vi "Nonlinear Curve Fit Intervals (Pearson option).vi"(0 "Y":dbl[](array[numeric]), 1 "confidence level":dbl=0.95, 2 "f(x,a)":T1, 3 "data":variant, 5 "X":dbl[](array[numeric]), 7 "Weight":dbl[](array[numeric]), 9 "best fit parameters":dbl[](array[numeric]), 11 "error in (no error)":errorcluster) -> (4 "Upper Bound":dbl[](array[numeric]), 6 "Lower Bound":dbl[](array[numeric]), 10 "delta best fit parameters":dbl[](array[numeric]), 15 "error out":errorcluster)   [LabVIEW 2021, in "Fits.lvlib"]
doc: "Calculates statistical intervals of the best nonlinear fit for a data set (<B>X</B>, <B>Y</B>)."
uses:
  <vilib>/gmath/NumericalOptimization/LM model function reference.ctl
  <vilib>/gmath/NumericalOptimization/LM_output select.ctl
  <vilib>/Analysis/baseanly.llb/Real A x B.vi
  <vilib>/gmath/statdist.llb/Student t Inverse CDF.vi
  <vilib>/Analysis/baseanly.llb/Real Inverse Matrix.vi
  Fits.lvlib
  <vilib>/Analysis/NI_AALPro.lvlib
  <vilib>/gmath/NI_Gmath.lvlib
  <vilib>/Analysis/NI_AALBase.lvlib
panel:
  # "see the License on the block diagram (Ctrl+E or Window:Show Block Diagram)"
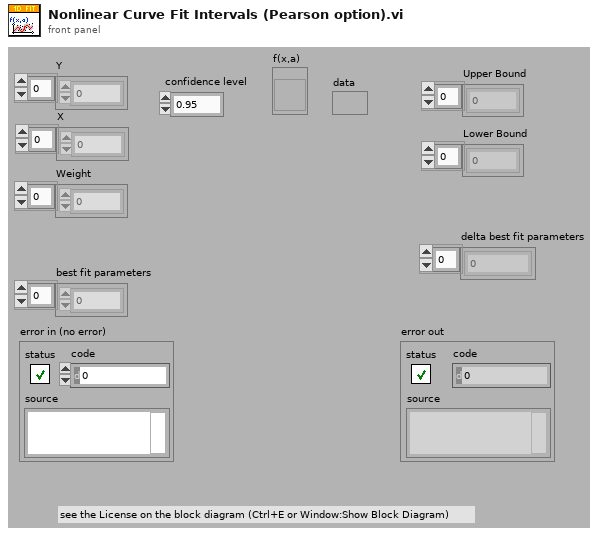
[diagram p1: front panel]
types:
  T1 = typedef "NI_Gmath.lvlib/LM model function reference.ctl" = refnum<vi>
  T2 = typedef "NI_Gmath.lvlib/LM_output select.ctl" = cluster{"model function":bool, "gradient":bool}
  T3 = typedef "NI_Matrix.lvlib/RealMatrix.ctl" = dbl[][]
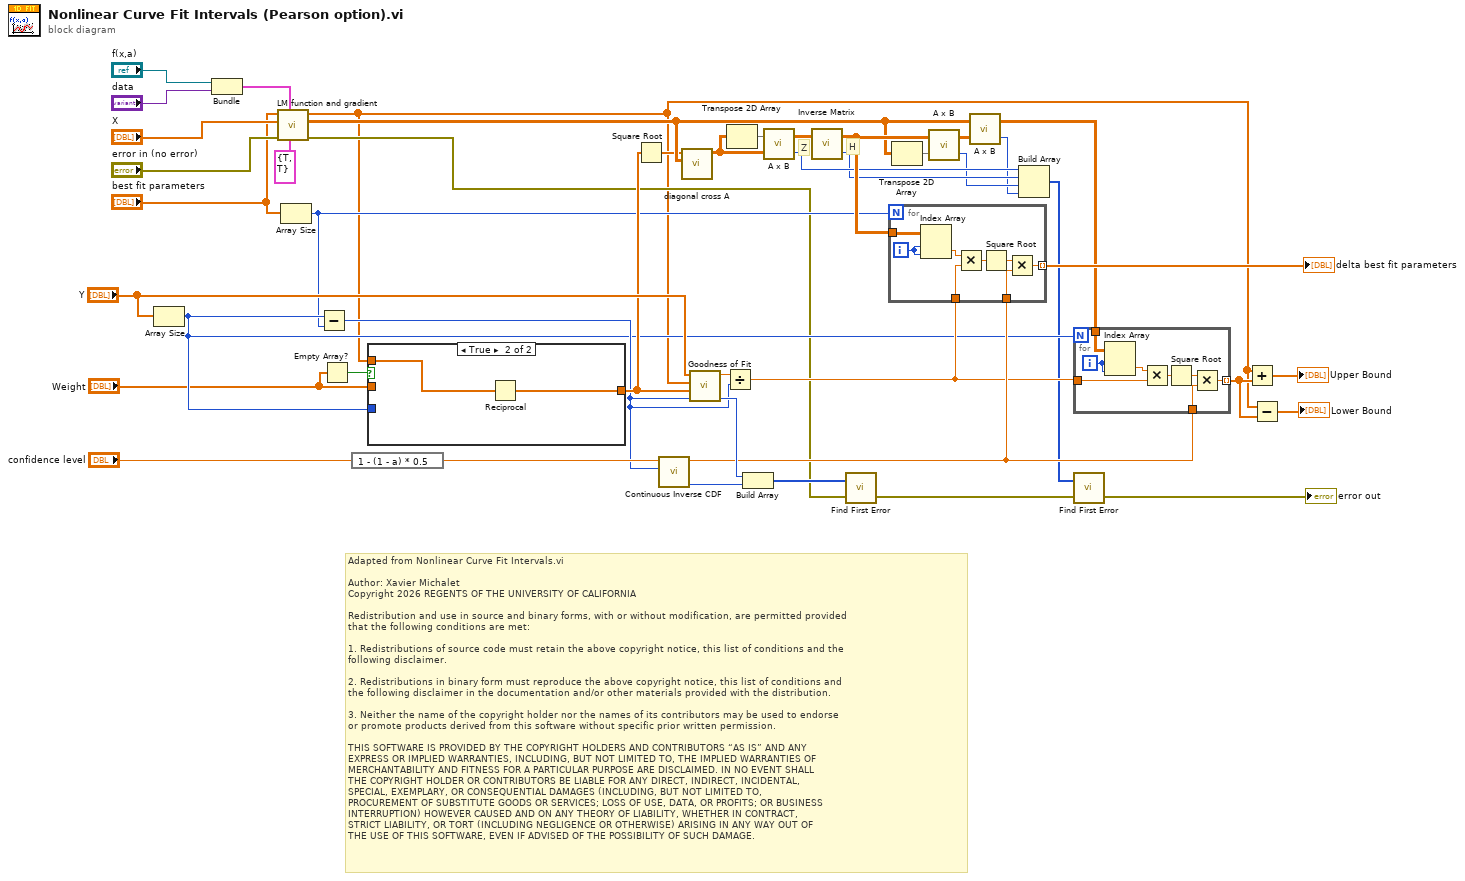
[diagram p0: block diagram]
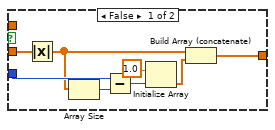
[diagram p2: hidden frame]
diagram:
  # "Adapted from Nonlinear Curve Fit Intervals.vi\n\nAuthor: Xavier Michalet\nCopyright 2026 REGENTS OF THE UNIVERSITY OF CALIFORNIA\n\nRedistribution and use in source and binary forms, with or without modification, are permitted provided\nthat the following conditions are met:\n\n1. Redistributions of source code must retain the above copyright notice, this list of conditions and the\nfollowing disclaimer.\n\n2. Redistributions in binary form must reproduce the above copyright notice, this list of conditions and\nthe following disclaimer in the documentation and/or other materials provided with the distribution.\n\n3. Neither the name of the copyright holder nor the names of its contributors may be used to endorse \nor promote products derived from this software without specific prior written permission.\n\nTHIS SOFTWARE IS PROVIDED BY THE COPYRIGHT HOLDERS AND CONTRIBUTORS “AS IS” AND ANY \nEXPRESS OR IMPLIED WARRANTIES, INCLUDING, BUT NOT LIMITED TO, THE IMPLIED WARRANTIES OF\nMERCHANTABILITY AND FITNESS FOR A PARTICULAR PURPOSE ARE DISCLAIMED. IN NO EVENT SHALL\nTHE COPYRIGHT HOLDER OR CONTRIBUTORS BE LIABLE FOR ANY DIRECT, INDIRECT, INCIDENTAL, \nSPECIAL, EXEMPLARY, OR CONSEQUENTIAL DAMAGES (INCLUDING, BUT NOT LIMITED TO, \nPROCUREMENT OF SUBSTITUTE GOODS OR SERVICES; LOSS OF USE, DATA, OR PROFITS; OR BUSINESS\nINTERRUPTION) HOWEVER CAUSED AND ON ANY THEORY OF LIABILITY, WHETHER IN CONTRACT, \nSTRICT LIABILITY, OR TORT (INCLUDING NEGLIGENCE OR OTHERWISE) ARISING IN ANY WAY OUT OF\nTHE USE OF THIS SOFTWARE, EVEN IF ADVISED OF THE POSSIBILITY OF SUCH DAMAGE."
  # "H"
  # "Z"
  n1 = Array Size(array="Y") -> (size(s)=w16:i32)
  n2 = Bundle("f(x,a)"="f(x,a)", "data"="data") -> (w40:cluster{"f(x,a)":T1, "data":variant})  [unwired: 1 in]
  n3 = call <vilib>:"LM function and gradient.vi"("output control"=T2 {"model function"=TRUE, "gradient"=TRUE}, "model function"=w40, "error in (no error)"="error in (no error)", "X"="X", "a"="best fit parameters") -> ("error out"=w7:errorcluster, "gradient"=w6:dbl[][], "f(X)"=w1:dbl[])  [unwired: 3 in, 1 out]
  n4 = Array Size(array="best fit parameters") -> (size(s)=w15:i32)
  n5 = Subtract(x=w16, y=w15) -> (x-y=w17:i32)
  n6 = Empty Array?(array="Weight") -> (empty?=w2:bool)
  n7 = expression code="1 - (1 - a) * 0.5"("confidence level") -> (w30:dbl)
  n8 = case shown="True" w2 {
    tunnel: "Weight" -> [w48 _]
    tunnel: [w47 w53] -> w18
    tunnel: w16 -> [w46 _]
    tunnel: w1 -> [_ w54]
    frame False {
      n9 = Absolute Value(x=w48) -> (abs(x)=w45:dbl[])
      n10 = Array Size(array=w45) -> (size(s)=w51:i32)
      n11 = Subtract(x=w46, y=w51) -> (x-y=w49:i32)
      n12 = Initialize Array(1.0, w49) -> (w50:dbl[])
      n13 = Build Array (concatenate)(w45, w50) -> (w47:dbl[])
    }
    frame True {
      n14 = Reciprocal(x=w54) -> (1/x=w53:dbl[])
    }
  }
  n15 = Square Root(x=w18) -> (sqrt(x)=w5:dbl[])
  n16 = call-poly <vilib>:"Continuous Inverse CDF.vi"("k degrees of freedom"=w17, "cdf(x)"=w30) -> ("error"=w29:i32, "x"=w24:dbl)  [unwired: 8 in]
  n17 = call <vilib>:"diagonal cross A.vi"("A"=w6, "diagonal"=w5) -> ("diagonalxA"=w4:T3)  [unwired: 9 in]
  n18 = call <vilib>:"Goodness of Fit.vi"("degree of freedom"=w17, "Weight"=w18, "Best Fit"=w1, "Y"="Y") -> ("error"=w32:i32, "SSE"=w33:dbl)  [unwired: 4 in, 2 out]
  n19 = Divide(x=w33, y=w17) -> (x/y=w20:dbl)
  n20 = Transpose 2D Array(2D array=w4) -> (transposed array=w36:T3)
  n21 = Build Array(w32, w29) -> (w31:i32[])
  n22 = call-poly <vilib>:"A x B.vi"("B"=w4, "A"=w36) -> ("error"=w14:i32, "A x B"=w35:T3)
  n23 = call-poly <vilib>:"Inverse Matrix.vi"("Input Matrix"=w35) -> ("error"=w13:i32, "Inverse Matrix"=w27:T3)  [unwired: 1 in]
  n24 = call <vilib>:"Find First Error.vi"("error in (no error)"=w7, "error codes"=w31) -> ("error out"=w10:errorcluster)  [unwired: 2 in, 1 out]
  n25 = for {
    N: w15 -> [_]
    tunnel: w27 -> [w62]
    tunnel: w24 -> [w55]
    tunnel: [w59] -> w44 mode=indexing
    tunnel: w20 -> [w56]
    i -> [w61]
    n26 = Index Array(array=w62, index (row)=w61, index (col)=w61) -> (element=w57:dbl)
    n27 = Multiply(x=w57, y=w56) -> (x*y=w60:dbl)
    n28 = Square Root(x=w60) -> (sqrt(x)=w58:dbl)
    n29 = Multiply(x=w58, y=w55) -> (x*y=w59:dbl)
  }
  "delta best fit parameters" <- w44
  n30 = Transpose 2D Array(2D array=w6) -> (transposed array=w28:dbl[][])
  n31 = call-poly <vilib>:"A x B.vi"("B"=w28, "A"=w27) -> ("error"=w12:i32, "A x B"=w26:T3)
  n32 = call-poly <vilib>:"A x B.vi"("B"=w26, "A"=w6) -> ("error"=w11:i32, "A x B"=w25:T3)
  n33 = Build Array(w14, w13, w12, w11) -> (w8:i32[])
  n34 = for {
    N: w16 -> [_]
    tunnel: w25 -> [w70]
    tunnel: w24 -> [w68]
    tunnel: [w67] -> w22 mode=indexing
    tunnel: w20 -> [w65]
    i -> [w63]
    n35 = Index Array(array=w70, index (row)=w63, index (col)=w63) -> (element=w66:dbl)
    n36 = Multiply(x=w66, y=w65) -> (x*y=w64:dbl)
    n37 = Square Root(x=w64) -> (sqrt(x)=w69:dbl)
    n38 = Multiply(x=w69, y=w68) -> (x*y=w67:dbl)
  }
  n39 = call <vilib>:"Find First Error.vi"("error in (no error)"=w10, "error codes"=w8) -> ("error out"=→"error out":errorcluster)  [unwired: 2 in, 1 out]
  n40 = Add(x=w1, y=w22) -> (x+y=→"Upper Bound":dbl[])
  n41 = Subtract(x=w1, y=w22) -> (x-y=→"Lower Bound":dbl[])
